vi "Size Select.vi"(11 "CtlRef":refnum<vi>) -> ()   [LabVIEW 2020, in "MDI ViewManager.lvlib"]
uses:
  MDI ViewManager.lvlib
panel:
  in  "OK Square":bool
  in  "Height":dbl
  in  "Widht":dbl
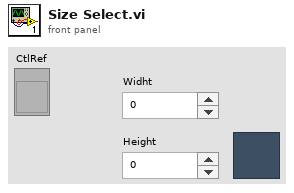
[diagram p1: front panel]
types:
  T1 = typedef "LVBoundsTypeDef.ctl" = cluster{"Width":u32, "Height":u32}
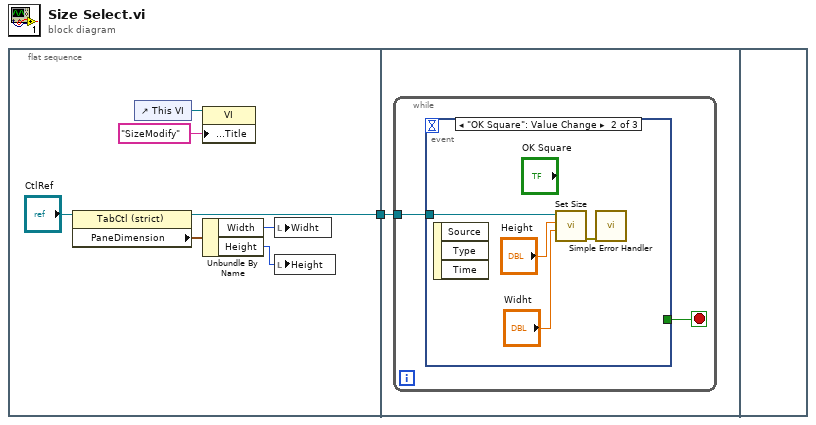
[diagram p0: block diagram]
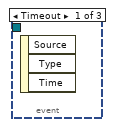
[diagram p2: hidden frame]
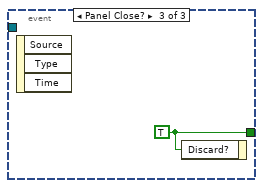
[diagram p3: hidden frame]
diagram:
  n1 = flat-sequence {
    tunnel: [w2] -> w1
    tunnel: w1 -> [w9]
    frame #0 {
      n2 = property class="TabCtl (strict)"(reference="CtlRef") -> (reference out=w2:refnum<vi>, "PaneDimension"=w3:T1)  [unwired: 1 in, 1 out]
      n3 = control-ref of="This VI"() -> (w6:refnum<vi>)
      n4 = property class="VI"(reference=w6, "Front Panel.Title"="SizeModify" ("VI Name")) -> ()  [unwired: 1 in, 2 out]
      n5 = Unbundle By Name(w3) -> ("Width"=w7:u32, "Height"=w8:u32)
      n6 = local write "Widht"(w7) -> ()
      n7 = local write "Height"(w8) -> ()
    }
    frame #1 {
      n8 = while {
        tunnel: w9 -> [w10]
        stop <- w11 stop-if-true
        n9 = event shown="[1] \"OK Square\": Value Change" {
          selector: _ -> [_ _ _]
          dyn-events: _ -> [_ _ _]
          timeout: _ -> [_ _ _]
          tunnel: [_ _ w16] -> w11
          tunnel: w10 -> [_ w15 _]
          event Timeout {
            n10 = event-data() -> ()  [unwired: 1 in, 3 out]
          }
          event "OK Square": Value Change {
            n11 = event-data() -> ()  [unwired: 1 in, 3 out]
            n12 = call "Set Size.vi"("Widht"="Widht", "Height"="Height", "TabControlRef in"=w15) -> ("error out"=w12:errorcluster)  [unwired: 7 in, 1 out]
            n13 = call <vilib>:"Simple Error Handler.vi"("error in (no error)"=w12) -> ()  [unwired: 4 in, 5 out]
          }
          event Panel Close? {
            w16 = TRUE ("Discard?")
            n14 = event-data() -> ()  [unwired: 1 in, 3 out]
            n15 = event-data("Discard?"=w16) -> ()  [unwired: 1 in, 1 out]
          }
        }
      }
    }
    frame #2 {
    }
  }
